vi "OAT Digital Tacho Process.vi"   [LabVIEW 2017, in "SoundVib_TachProcess.lvlib"]
doc: "Locates tachometer pulse positions in the digital tachometer signal and calculates the rotational speed of a device. Wire data to the <B>digital tacho info</B> input to determine the polymorphic instance to use or manually select the instance."
uses:
  <vilib>/addons/Sound and Vibration/Order Analysis/Tach Process/SoundVib_TachProcess.lvlib
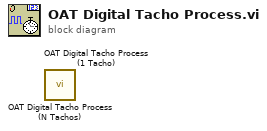
[diagram p0: block diagram]
diagram:
  n1 = call <vilib>:"OAT Digital Tacho Process (N Tachos).vi"() -> ()  [unwired: 12 in, 4 out]
  n2 = call <vilib>:"OAT Digital Tacho Process (1 Tacho).vi"() -> ()  [unwired: 12 in, 4 out]
